vi "change VI visibility.vi"(8 "error in (no error)":errorcluster, 11 "State (hidden)":T1(ring)=enum."Hidden") -> (0 "error out":errorcluster)   [LabVIEW 2021, in "AF Utils.lvlib"]
doc: "Change the referenced VIs state to that selected (hidden default)"
uses:
  AF Utils.lvlib
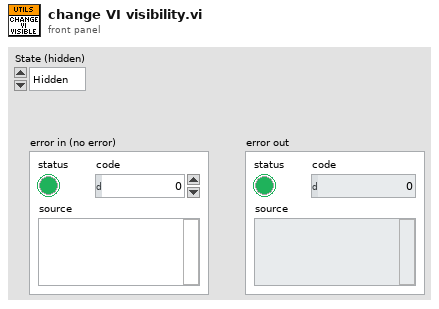
[diagram p1: front panel]
types:
  T1 = enum32{"Invalid", "Standard", "Closed", "Hidden", "Minimized", "Maximized"}
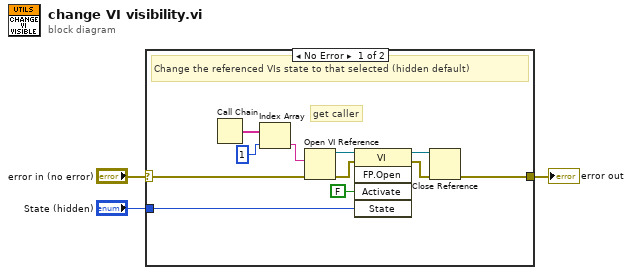
[diagram p0: block diagram]
diagram:
  n1 = case shown="No Error" "error in (no error)" {
    selector: "error in (no error)" -> [w4 w15]
    tunnel: [w14 w15] -> w3
    tunnel: "State (hidden)" -> [w11 _]
    frame No Error {
      # "get caller"
      # "Change the referenced VIs state to that selected (hidden default)"
      n2 = Call Chain() -> (call chain=w7:string[])
      n3 = Index Array(array=w7, index=1) -> (element=w5:string)
      n4 = Open VI Reference(vi path=w5, error in (no error)=w4) -> (vi reference=w8:refnum<vi>, error out=w9:errorcluster)  [unwired: 4 in]
      n5 = invoke class="VI" method="FP.Open"(reference=w8, error in=w9, "Activate"=FALSE ("Activate?"), "State"=w11) -> (reference out=w12:refnum<vi>, error out=w13:errorcluster)  [unwired: 1 in, 3 out]
      n6 = Close Reference(reference=w12, error in (no error)=w13) -> (error out=w14:errorcluster)
    }
    frame Error {
    }
  }
  "error out" <- w3
